vi "terminate.vi"(8 "error in (no error)":errorcluster, 11 "reference in":refnum<class "Master Controller.lvclass">) -> (0 "error out":errorcluster, 3 "reference out":refnum<class "Master Controller.lvclass">)   [LabVIEW 2015, in "Master Controller.lvclass"]
uses:
  Master Controller.lvclass
  GUI/GUI Controller_llb/GUI Controller.lvclass
  File Controller_llb/File Controller.lvclass
  Subject Controller_llb/Subject Controller.lvclass
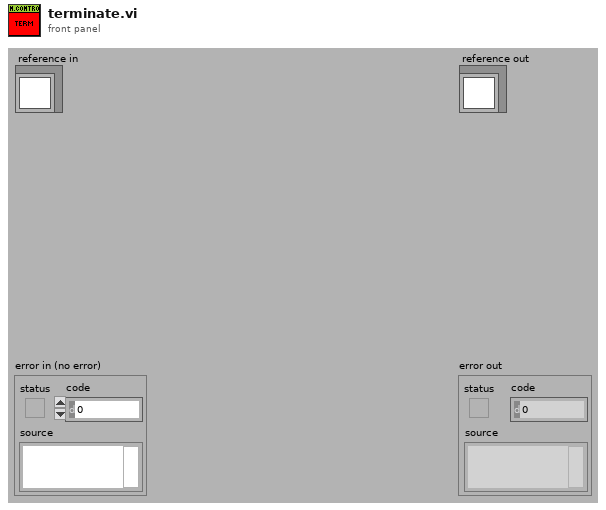
[diagram p1: front panel]
types:
  T1 = typedef "Master Controller.lvclass/ObjectAttributesRef.ctl" = refnum<data-value>
  T2 = typedef "Master Controller.lvclass/ObjectAttributes.ctl" = cluster{"MyAttribute":dbl, "gui_controller_ref":refnum<class "GUI Controller.lvclass">, "file_controller_ref":refnum<class "File Controller.lvclass">, "subject_controller_ref":refnum<class "Subject Controller.lvclass">}
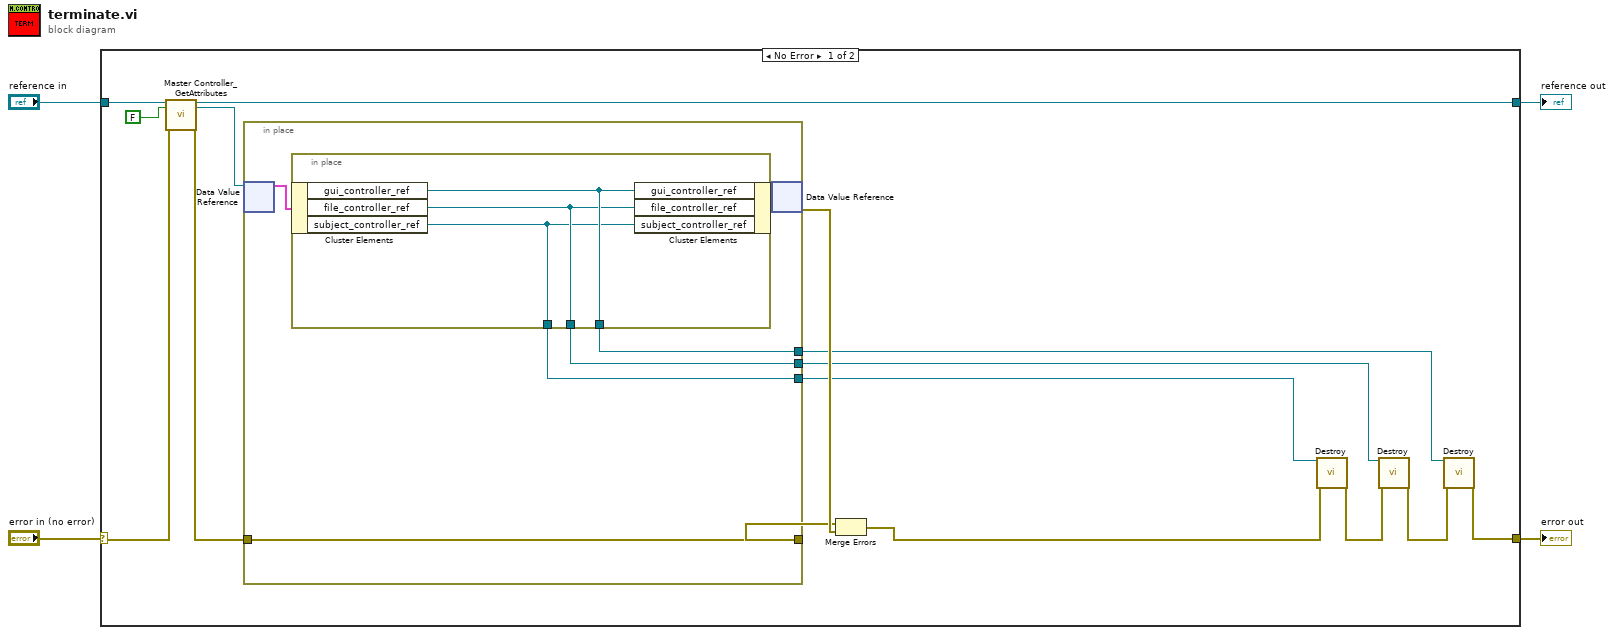
[diagram p0: block diagram]
diagram:
  n1 = case shown="No Error" "error in (no error)" {
    selector: "error in (no error)" -> [w15 w30]
    tunnel: [w10 w30] -> w3
    tunnel: [w13 w29] -> w1
    tunnel: "reference in" -> [w17 w29]
    frame No Error {
      n2 = call "Master Controller_GetAttributes.vi"("reference in"=w17, "return data? (T)"=FALSE, "error in (no error)"=w15) -> ("reference out"=w13:refnum<class "Master Controller.lvclass">, "attributes ref"=w12:T1, "error out"=w14:errorcluster)  [unwired: 13 in, 1 out]
      n3 = in-place {
        in-place-border: w14 -> [w23]
        in-place-border: [w23] -> w18
        in-place-border: [w22] -> w11
        in-place-border: [w21] -> w9
        in-place-border: [w20] -> w7
        n4 = in-place-dvr #1(w12) -> (w24:T2)  [unwired: 1 out]
        n5 = in-place {
          in-place-border: [w28] -> w22
          in-place-border: [w27] -> w21
          in-place-border: [w26] -> w20
          n6 = in-place-cluster #2(w24) -> ("gui_controller_ref"=w28:refnum<class "GUI Controller.lvclass">, "file_controller_ref"=w27:refnum<class "File Controller.lvclass">, "subject_controller_ref"=w26:refnum<class "Subject Controller.lvclass">)
          n7 = in-place-cluster #2("gui_controller_ref"=w28, "file_controller_ref"=w27, "subject_controller_ref"=w26) -> (w25:T2)
        }
        n8 = in-place-dvr #1(w25) -> (w19:errorcluster)  [unwired: 1 out]
      }
      n9 = Merge Errors(w18, w19) -> (w6:errorcluster)
      n10 = call-dynamic "Destroy.vi"("reference in"=w7, "error in (no error)"=w6) -> ("error out"=w5:errorcluster)  [unwired: 16 in, 1 out]
      n11 = call-dynamic "Destroy.vi"("reference in"=w9, "error in (no error)"=w5) -> ("error out"=w8:errorcluster)  [unwired: 16 in, 1 out]
      n12 = call-dynamic "Destroy.vi"("reference in"=w11, "error in (no error)"=w8) -> ("error out"=w10:errorcluster)  [unwired: 16 in, 1 out]
    }
    frame Error {
    }
  }
  "error out" <- w3
  "reference out" <- w1
